vi "SRingBlockTrig.vi"(1 "channel 1, 2 or 3":u8=1) -> (0 "Boolesch":bool)   [LabVIEW 2015]
uses:
  ESLSCDLL.dll
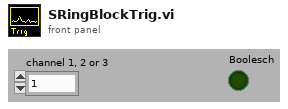
[diagram p1: front panel]
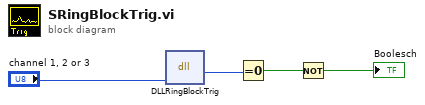
[diagram p0: block diagram]
diagram:
  n1 = dll-call lib="C:/ENTW/PCIE/64bit/lv64/1cam/board.vis/ESLSCDLL.dll" fn="DLLRingBlockTrig" ("lwlscdll.dll:DLLTempGood")("ch"="channel 1, 2 or 3") -> ("Rückgabetyp"=w3:u8)  [unwired: 4 in, 2 out]
  n2 = Equal To 0?(x=w3) -> (x = 0?=w2:bool)
  n3 = Not(x=w2) -> (.not. x?=→"Boolesch":bool)
